vi "Set payload length bytes.vi"(8 "error in (no error)":errorcluster, 10 "payload length bytes":i32=48, 11 "niDTS WLAN Dut in":refnum<class "niDTS WLAN Dut.lvclass">) -> (0 "error out":errorcluster, 3 "niDTS WLAN Dut out":refnum<class "niDTS WLAN Dut.lvclass">)   [LabVIEW 2015, in "niDTS WLAN.lvlib" / "niDTS WLAN Dut.lvclass"]
uses:
  niDTS WLAN Dut.lvclass
  niDTS WLAN Dut.lvclass/niDTS WLAN Dut.ctl
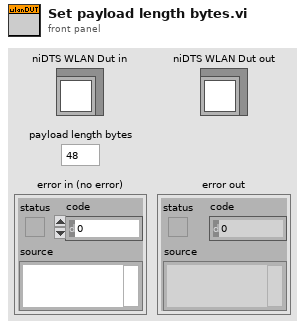
[diagram p1: front panel]
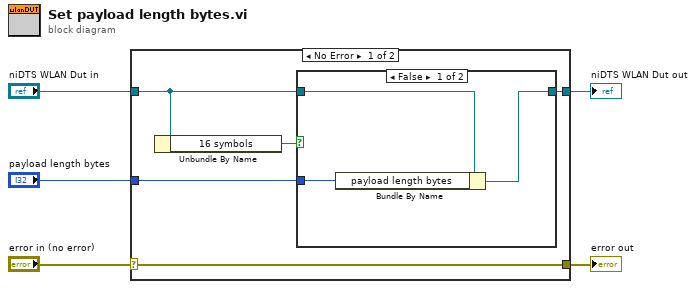
[diagram p0: block diagram]
diagram:
  n1 = case shown="No Error" "error in (no error)" {
    selector: "error in (no error)" -> [w10 w15]
    tunnel: [w10 w15] -> w4
    tunnel: [w9 w16] -> w2
    tunnel: "niDTS WLAN Dut in" -> [w7 w16]
    tunnel: "payload length bytes" -> [w8 _]
    frame No Error {
      n2 = Unbundle By Name(w7) -> ("16 symbols"=w6:bool)
      n3 = case shown="False" w6 {
        tunnel: [w13 w14] -> w9
        tunnel: w8 -> [w12 _]
        tunnel: w7 -> [w11 w14]
        frame False {
          n4 = Bundle By Name(cluster=w11, "payload length bytes"=w12) -> (w13:refnum<class "niDTS WLAN Dut.lvclass">)
        }
        frame True {
          # "Do Nothing."
        }
      }
    }
    frame Error {
    }
  }
  "error out" <- w4
  "niDTS WLAN Dut out" <- w2
